vi "MeasureEQE_ActiveX.vi"(6 "Skip?":bool, 8 "error in (no error)":errorcluster, 9 "Save data file path":string, 10 "Scan settings":T1={"J-V scan"=TRUE, "J-t scan"=FALSE, "Min voltage (V)"=0.0, "Max voltage (V)"=1.4, "Step (V)"=0.01, "Measurement delay (ms)"=10.0, "1st scan FB-SC"=TRUE, "Inverted structure"=FALSE, "Stabilisation time (s)"=0.0, "Stabilisation mode"=0, "Stabilisation value (V or A) "=0.0, "Step time (s)"=1.0, "Integration time"=0, "Repeat light scans"=FALSE, "Stabilisation in the dark?"=FALSE, "J-t Min (V)"=0.0, "J-t Max (V)"=1.4, "J-t Step (V)"=0.01, "Max. power stabilisation"=FALSE, "J-t 1st scan FB-SC"=TRUE, "J-t Inverted structure"=FALSE, "Max power tracking"=FALSE, "Vmp (V)"=0.7, "Total stabilisation time (s)"=100.0, "J-t best pixel only"=0, "Max power best pixel only"=0, "Vmp from J-V scan"=FALSE, "Intensity dependence"=FALSE, "P dep best pixel only"=0, "External quantum efficiency"=FALSE, "EQE best pixel only"=0, "WL min (nm)"=300.0, "WL max (nm)"=900.0, "WL step (nm)"=5.0, "Wait (ms)"=100.0, "No. of repeat scans"=2.0, "Only repeat for best pixel"=0, "Chopper Freq.  (Hz)"=90.0, "Time Constant (s)"=2.0, "Stabilisation time step (s)"=1.0, "Illumination conditions"=2, "Scan rate min (V/s)"=0.1, "Scan rate max (V/s)"=1.0, "No. of scan rate steps"=1.0, "Scan rate voltage step priority"=FALSE, "Scan rate measurement delay priority"=FALSE, "J-t Illumination conditions"=0, "White bias  (no. of suns)"=200.0, "Max P stab. Specific voltage"=FALSE} {"J-t Illumination conditions" items=["Light only", "Dark only", "Light then dark", "Dark then light"]; "No. of scan rate steps" min=1.0 step=1.0; "Illumination conditions" items=["Light only", "Dark only", "Light then dark", "Dark then light", "Light then dark then light", "Dark then light then dark"]; "Time Constant (s)" items=["0.003", "0.01", "0.03", "0.1", "0.3", "1", "3", "10", "30", "100"]; "Only repeat for best pixel" items=["only for best pixel", "for best 2 pixels", "for best 3 pixels", "for best 4 pixels", "for best 5 pixels", "for best 6 pixels", "for best 7 pixels", "for all pixels"]; "No. of repeat scans" min=1.0 step=1.0; "EQE best pixel only" items=["only the best pixel", "the best 2 pixel", "the best 3 pixel", "the best 4 pixel", "the best 5 pixel", "the best 6 pixel", "the best 7 pixel", "all pixels"]; "P dep best pixel only" items=["only the best pixel", "the best 2 pixels", "the best 3 pixels", "the best 4 pixels", "the best 5 pixels", "the best 6 pixels", "the best 7 pixels", "all pixels"]; "Max power best pixel only" items=["only the best pixel", "the best 2 pixels", "the best 3 pixels", "the best 4 pixels", "the best 5 pixels", "the best 6 pixels", "the best 7 pixels", "all pixels"]; "J-t best pixel only" items=["only the best pixel", "the best 2 pixels", "the best 3 pixels", "the best 4 pixels", "the best 5 pixels", "the best 6 pixels", "the best 7 pixels", "all pixels"]; "Integration time" items=["Fast", "Normal", "High Accuracy"]; "Stabilisation mode" items=["V", "I"]; "Measurement delay (ms)" min=10.0}) -> (0 "error out":errorcluster, 1 "Min WL (nm)":string, 2 "Max WL (nm)":string, 3 "EQE data file path":path)   [LabVIEW 2011]
uses:
  TypeDefs/Scan settings.ctl
  TypeDefs/Settings Boolean.ctl
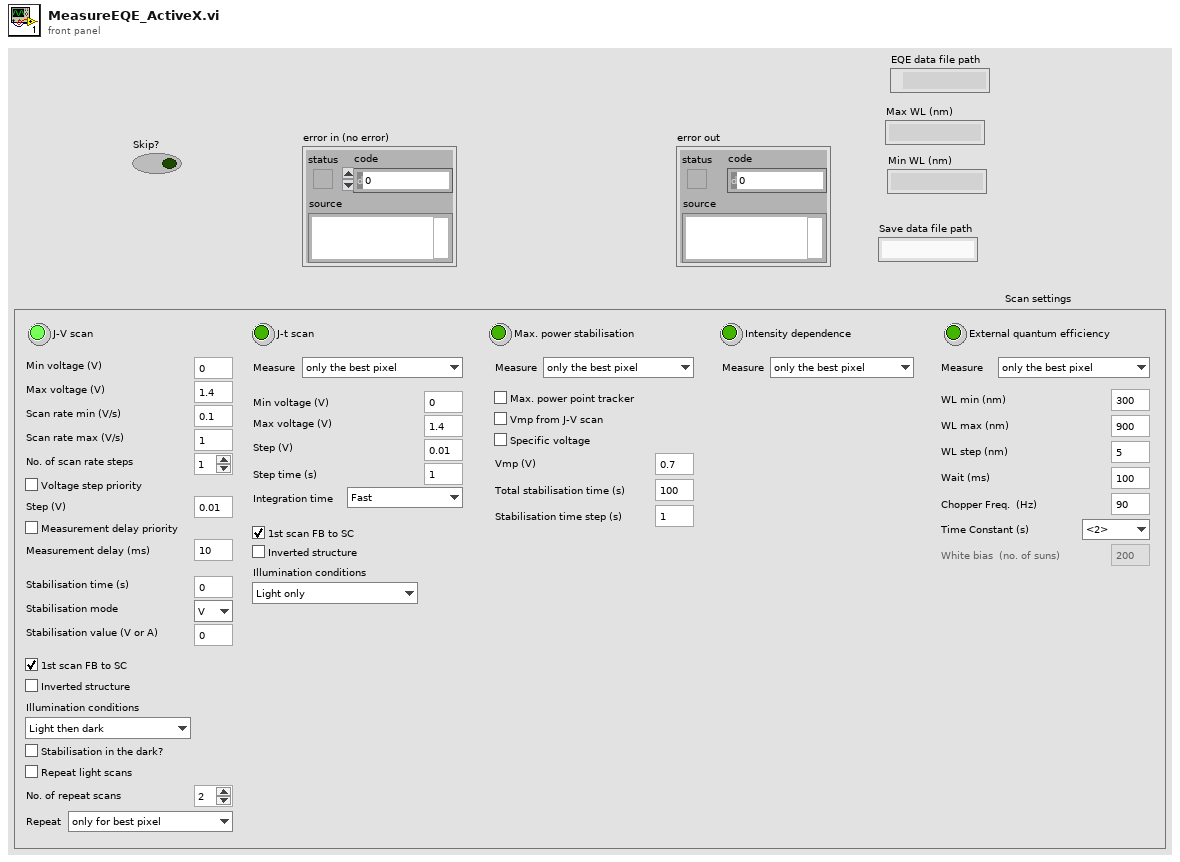
[diagram p1: front panel]
types:
  T1 = typedef "Scan settings.ctl" = cluster{"J-V scan":T2, "J-t scan":bool, "Min voltage (V)":dbl, "Max voltage (V)":dbl, "Step (V)":dbl, "Measurement delay (ms)":dbl, "1st scan FB-SC":bool, "Inverted structure":bool, "Stabilisation time (s)":dbl, "Stabilisation mode":u16, "Stabilisation value (V or A) ":dbl, "Step time (s)":dbl, "Integration time":u16, "Repeat light scans":bool, "Stabilisation in the dark?":bool, "J-t Min (V)":dbl, "J-t Max (V)":dbl, "J-t Step (V)":dbl, "Max. power stabilisation":bool, "J-t 1st scan FB-SC":bool, "J-t Inverted structure":bool, "Max power tracking":bool, "Vmp (V)":dbl, "Total stabilisation time (s)":dbl, "J-t best pixel only":u16, "Max power best pixel only":u16, "Vmp from J-V scan":bool, "Intensity dependence":bool, "P dep best pixel only":u16, "External quantum efficiency":bool, "EQE best pixel only":u16, "WL min (nm)":dbl, "WL max (nm)":dbl, "WL step (nm)":dbl, "Wait (ms)":dbl, "No. of repeat scans":dbl, "Only repeat for best pixel":u16, "Chopper Freq.  (Hz)":dbl, "Time Constant (s)":dbl, "Stabilisation time step (s)":dbl, "Illumination conditions":u16, "Scan rate min (V/s)":dbl, "Scan rate max (V/s)":dbl, "No. of scan rate steps":dbl, "Scan rate voltage step priority":bool, "Scan rate measurement delay priority":bool, "J-t Illumination conditions":u16, "White bias  (no. of suns)":dbl, "Max P stab. Specific voltage":bool}
  T2 = typedef "Settings Boolean.ctl" = bool
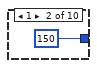
[diagram p2: hidden frame]
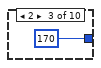
[diagram p3: hidden frame]
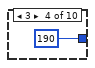
[diagram p4: hidden frame]
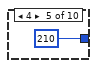
[diagram p5: hidden frame]
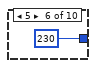
[diagram p6: hidden frame]
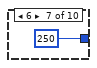
[diagram p7: hidden frame]
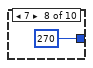
[diagram p8: hidden frame]
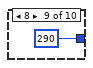
[diagram p9: hidden frame]
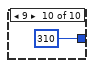
[diagram p10: hidden frame]
diagram:
  n1 = case shown="False" "Skip?" {
    tunnel: "error in (no error)" -> [w273 w285]
    tunnel: [w4 w285] -> w2
    frame False {
      w13 = 2000.0  # Buffer (ms)
      w14 = 11000.0  # Grating change time (ms)
      w17 = 2000.0  # Filter change time (ms)
      w18 = 22000.0  # initialisation time (ms)
      w21 = 1150.0  # time to change wl and measure (ms)
      # "click \"Clear graph\""
      # "click \"Ok\""
      # "Save file"
      # "click \"Save scan data\""
      # "click \"File\""
      # "click \"Take a simple wavelength scan\""
      # "click \"Scan\""
      # "Click \"OK\""
      # "Set wait"
      # "Set wavlength step"
      # "Set end wavlength"
      # "Set start wavlength"
      # "click \"Click Setup Scan Wavelength Parameters\""
      # "click \"Scan\""
      # "click \"OK\""
      # "click \"AC\""
      # "click \"Ref Type\""
      # "set chopper frequency (Hz)"
      # "choose time constant"
      # "click \"Time Constant\""
      # "click \"CHANNEL 2\""
      # "click \"Channel Setup\""
      # "click \"Setup Parameters\""
      # "click \"Detector\""
      n2 = Automation Open(error in (no error)=w273, Automation Refnum=refnum<k7> refnum ("AutoItX3Lib.IAutoItX3")) -> (Automation Refnum=w238:refnum<k7>, error out=w237:errorcluster)  [unwired: 2 in]
      n3 = invoke class="IAutoItX3" method="WinActivate"(reference=w238, error in=w237, "strTitle"="Newport Oriel Tracq Basic Version 6.2", "strText"="") -> (reference out=w272:refnum<k7>, error out=w265:errorcluster)  [unwired: 1 in, 3 out]
      n4 = invoke class="IAutoItX3" method="WinWaitActive"(reference=w272, error in=w265, "strTitle"="Newport Oriel Tracq Basic Version 6.2", "strText"="", "nTimeout"=2000) -> (reference out=w266:refnum<k7>, error out=w264:errorcluster)  [unwired: 1 in, 4 out]
      n5 = invoke class="IAutoItX3" method="MouseClick"(reference=w266, error in=w264, "strButton"="primary", "nX"=250, "nY"=40, "nClicks"=1) -> (reference out=w258:refnum<k7>, error out=w257:errorcluster)  [unwired: 2 in, 6 out]
      n6 = invoke class="IAutoItX3" method="Sleep"(reference=w258, error in=w257, "nMilliseconds"=100) -> (reference out=w252:refnum<k7>, error out=w251:errorcluster)  [unwired: 1 in, 2 out]
      n7 = invoke class="IAutoItX3" method="MouseClick"(reference=w252, error in=w251, "strButton"="primary", "nX"=290, "nY"=90, "nClicks"=1) -> (reference out=w247:refnum<k7>, error out=w246:errorcluster)  [unwired: 2 in, 6 out]
      n8 = invoke class="IAutoItX3" method="WinWaitActive"(reference=w247, error in=w246, "strTitle"="Merlin Setup", "strText"="", "nTimeout"=5000) -> (reference out=w232:refnum<k7>, error out=w231:errorcluster)  [unwired: 1 in, 4 out]
      n9 = invoke class="IAutoItX3" method="MouseClick"(reference=w232, error in=w231, "strButton"="primary", "nX"=450, "nY"=70, "nClicks"=1) -> (reference out=w223:refnum<k7>, error out=w222:errorcluster)  [unwired: 2 in, 6 out]
      n10 = invoke class="IAutoItX3" method="Sleep"(reference=w223, error in=w222, "nMilliseconds"=100) -> (reference out=w225:refnum<k7>, error out=w224:errorcluster)  [unwired: 1 in, 2 out]
      n11 = invoke class="IAutoItX3" method="MouseClick"(reference=w225, error in=w224, "strButton"="primary", "nX"=365, "nY"=140, "nClicks"=1) -> (reference out=w214:refnum<k7>, error out=w213:errorcluster)  [unwired: 2 in, 6 out]
      n12 = invoke class="IAutoItX3" method="Sleep"(reference=w214, error in=w213, "nMilliseconds"=100) -> (reference out=w216:refnum<k7>, error out=w215:errorcluster)  [unwired: 1 in, 2 out]
      n13 = Unbundle By Name("Scan settings") -> ("WL min (nm)"=w11:dbl, "WL max (nm)"=w12:dbl, "WL step (nm)"=w10:dbl, "Wait (ms)"=w9:dbl, "Chopper Freq.  (Hz)"=w30:dbl, "Time Constant (s)"=w33:dbl)
      n14 = invoke class="IAutoItX3" method="MouseClick"(reference=w216, error in=w215, "strButton"="primary", "nX"=865, "nY"=310, "nClicks"=1) -> (reference out=w211:refnum<k7>, error out=w210:errorcluster)  [unwired: 2 in, 6 out]
      n15 = case shown="0, Default" w33 {
        tunnel: [130 150 170 190 210 230 250 270 290 310] -> w31
        frame 0, Default {
        }
        frame 1 {
        }
        frame 2 {
        }
        frame 3 {
        }
        frame 4 {
        }
        frame 5 {
        }
        frame 6 {
        }
        frame 7 {
        }
        frame 8 {
        }
        frame 9 {
        }
      }
      n16 = invoke class="IAutoItX3" method="Sleep"(reference=w211, error in=w210, "nMilliseconds"=100) -> (reference out=w204:refnum<k7>, error out=w203:errorcluster)  [unwired: 1 in, 2 out]
      n17 = invoke class="IAutoItX3" method="MouseClick"(reference=w204, error in=w203, "strButton"="primary", "nX"=865, "nY"=w31, "nClicks"=1) -> (reference out=w206:refnum<k7>, error out=w205:errorcluster)  [unwired: 2 in, 6 out]
      n18 = Number To Fractional String(number=w11) -> (F-format string=w28:string)  [unwired: 3 in]
      "Min WL (nm)" <- w28
      n19 = Number To Fractional String(number=w12) -> (F-format string=w27:string)  [unwired: 3 in]
      "Max WL (nm)" <- w27
      n20 = Number To Fractional String(number=w10) -> (F-format string=w26:string)  [unwired: 3 in]
      n21 = Number To Fractional String(number=w9) -> (F-format string=w25:string)  [unwired: 3 in]
      n22 = Number To Fractional String(number=w30) -> (F-format string=w29:string)  [unwired: 3 in]
      n23 = invoke class="IAutoItX3" method="Sleep"(reference=w206, error in=w205, "nMilliseconds"=100) -> (reference out=w202:refnum<k7>, error out=w201:errorcluster)  [unwired: 1 in, 2 out]
      n24 = Subtract(x=w12, y=w11) -> (x-y=w24:dbl)
      n25 = Divide(x=w24, y=w10) -> (x/y=w23:dbl)
      n26 = Increment(x=w23) -> (x+1=w22:dbl)
      n27 = Add(x=w9, y=w21) -> (x+y=w20:dbl)
      n28 = Multiply(x=w22, y=w20) -> (x*y=w19:dbl)
      n29 = invoke class="IAutoItX3" method="MouseClickDrag"(reference=w202, error in=w201, "strButton"="primary", "nX1"=870 ("nX"), "nY1"=370 ("nY"), "nX2"=825 ("nClicks"), "nY2"=370 ("nClicks")) -> (reference out=w240:refnum<k7>, error out=w239:errorcluster)  [unwired: 2 in, 7 out]
      n30 = Multiply(x=w17, y=2.0) -> (x*y=w15:dbl)
      n31 = invoke class="IAutoItX3" method="Send"(reference=w240, error in=w239, "strSendText"=w29) -> (reference out=w193:refnum<k7>, error out=w192:errorcluster)  [unwired: 2 in, 3 out]
      n32 = Compound Arithmetic op=ADD(w19, w18, w15, w14, w13) -> (w8:dbl)
      n33 = invoke class="IAutoItX3" method="Sleep"(reference=w193, error in=w192, "nMilliseconds"=100) -> (reference out=w195:refnum<k7>, error out=w194:errorcluster)  [unwired: 1 in, 2 out]
      n34 = To Long Integer(number=w8) -> (32bit integer=w7:i32)
      n35 = invoke class="IAutoItX3" method="MouseClick"(reference=w195, error in=w194, "strButton"="primary", "nX"=910, "nY"=695, "nClicks"=1) -> (reference out=w184:refnum<k7>, error out=w183:errorcluster)  [unwired: 2 in, 6 out]
      n36 = invoke class="IAutoItX3" method="Sleep"(reference=w184, error in=w183, "nMilliseconds"=100) -> (reference out=w186:refnum<k7>, error out=w185:errorcluster)  [unwired: 1 in, 2 out]
      n37 = invoke class="IAutoItX3" method="MouseClick"(reference=w186, error in=w185, "strButton"="primary", "nX"=830, "nY"=740, "nClicks"=1) -> (reference out=w175:refnum<k7>, error out=w174:errorcluster)  [unwired: 2 in, 6 out]
      n38 = invoke class="IAutoItX3" method="Sleep"(reference=w175, error in=w174, "nMilliseconds"=100) -> (reference out=w177:refnum<k7>, error out=w176:errorcluster)  [unwired: 1 in, 2 out]
      n39 = invoke class="IAutoItX3" method="MouseClick"(reference=w177, error in=w176, "strButton"="primary", "nX"=1125, "nY"=75, "nClicks"=1) -> (reference out=w170:refnum<k7>, error out=w169:errorcluster)  [unwired: 2 in, 6 out]
      n40 = invoke class="IAutoItX3" method="WinWaitActive"(reference=w170, error in=w169, "strTitle"="Newport Oriel Tracq Basic Version 6.2", "strText"="", "nTimeout"=10000) -> (reference out=w155:refnum<k7>, error out=w154:errorcluster)  [unwired: 1 in, 4 out]
      n41 = invoke class="IAutoItX3" method="MouseClick"(reference=w155, error in=w154, "strButton"="primary", "nX"=50, "nY"=35, "nClicks"=1) -> (reference out=w157:refnum<k7>, error out=w156:errorcluster)  [unwired: 2 in, 6 out]
      n42 = invoke class="IAutoItX3" method="Sleep"(reference=w157, error in=w156, "nMilliseconds"=100) -> (reference out=w159:refnum<k7>, error out=w158:errorcluster)  [unwired: 1 in, 2 out]
      n43 = invoke class="IAutoItX3" method="MouseClick"(reference=w159, error in=w158, "strButton"="primary", "nX"=45, "nY"=55, "nClicks"=1) -> (reference out=w150:refnum<k7>, error out=w149:errorcluster)  [unwired: 2 in, 6 out]
      n44 = invoke class="IAutoItX3" method="WinWaitActive"(reference=w150, error in=w149, "strTitle"="Enter Scan Parameters", "strText"="", "nTimeout"=2000) -> (reference out=w141:refnum<k7>, error out=w140:errorcluster)  [unwired: 1 in, 4 out]
      n45 = invoke class="IAutoItX3" method="MouseClickDrag"(reference=w141, error in=w140, "strButton"="primary", "nX1"=675 ("nX"), "nY1"=470 ("nY"), "nX2"=600 ("nClicks"), "nY2"=470 ("nClicks")) -> (reference out=w143:refnum<k7>, error out=w142:errorcluster)  [unwired: 2 in, 7 out]
      n46 = invoke class="IAutoItX3" method="Send"(reference=w143, error in=w142, "strSendText"=w28) -> (reference out=w132:refnum<k7>, error out=w131:errorcluster)  [unwired: 2 in, 3 out]
      n47 = invoke class="IAutoItX3" method="MouseClickDrag"(reference=w132, error in=w131, "strButton"="primary", "nX1"=675 ("nX"), "nY1"=515 ("nY"), "nX2"=600 ("nClicks"), "nY2"=515 ("nClicks")) -> (reference out=w134:refnum<k7>, error out=w133:errorcluster)  [unwired: 2 in, 7 out]
      n48 = invoke class="IAutoItX3" method="Send"(reference=w134, error in=w133, "strSendText"=w27) -> (reference out=w123:refnum<k7>, error out=w122:errorcluster)  [unwired: 2 in, 3 out]
      n49 = invoke class="IAutoItX3" method="MouseClickDrag"(reference=w123, error in=w122, "strButton"="primary", "nX1"=675 ("nX"), "nY1"=560 ("nY"), "nX2"=600 ("nClicks"), "nY2"=560 ("nClicks")) -> (reference out=w125:refnum<k7>, error out=w124:errorcluster)  [unwired: 2 in, 7 out]
      n50 = invoke class="IAutoItX3" method="Send"(reference=w125, error in=w124, "strSendText"=w26) -> (reference out=w114:refnum<k7>, error out=w113:errorcluster)  [unwired: 2 in, 3 out]
      n51 = invoke class="IAutoItX3" method="MouseClickDrag"(reference=w114, error in=w113, "strButton"="primary", "nX1"=675 ("nX"), "nY1"=600 ("nY"), "nX2"=600 ("nClicks"), "nY2"=600 ("nClicks")) -> (reference out=w116:refnum<k7>, error out=w115:errorcluster)  [unwired: 2 in, 7 out]
      n52 = invoke class="IAutoItX3" method="Send"(reference=w116, error in=w115, "strSendText"=w25) -> (reference out=w103:refnum<k7>, error out=w102:errorcluster)  [unwired: 2 in, 3 out]
      n53 = invoke class="IAutoItX3" method="MouseClick"(reference=w103, error in=w102, "strButton"="primary", "nX"=801, "nY"=425, "nClicks"=1) -> (reference out=w105:refnum<k7>, error out=w104:errorcluster)  [unwired: 2 in, 6 out]
      n54 = invoke class="IAutoItX3" method="WinWaitActive"(reference=w105, error in=w104, "strTitle"="Newport Oriel Tracq Basic Version 6.2", "strText"="", "nTimeout"=2000) -> (reference out=w94:refnum<k7>, error out=w93:errorcluster)  [unwired: 1 in, 4 out]
      n55 = invoke class="IAutoItX3" method="MouseClick"(reference=w94, error in=w93, "strButton"="primary", "nX"=50, "nY"=35, "nClicks"=1) -> (reference out=w96:refnum<k7>, error out=w95:errorcluster)  [unwired: 2 in, 6 out]
      n56 = invoke class="IAutoItX3" method="Sleep"(reference=w96, error in=w95, "nMilliseconds"=100) -> (reference out=w86:refnum<k7>, error out=w85:errorcluster)  [unwired: 1 in, 2 out]
      n57 = invoke class="IAutoItX3" method="MouseClick"(reference=w86, error in=w85, "strButton"="primary", "nX"=60, "nY"=80, "nClicks"=1) -> (reference out=w88:refnum<k7>, error out=w87:errorcluster)  [unwired: 2 in, 6 out]
      n58 = invoke class="IAutoItX3" method="Sleep"(reference=w88, error in=w87, "nMilliseconds"=w7) -> (reference out=w71:refnum<k7>, error out=w70:errorcluster)  [unwired: 1 in, 2 out]
      n59 = invoke class="IAutoItX3" method="MouseClick"(reference=w71, error in=w70, "strButton"="primary", "nX"=15, "nY"=35, "nClicks"=1) -> (reference out=w79:refnum<k7>, error out=w78:errorcluster)  [unwired: 2 in, 6 out]
      n60 = invoke class="IAutoItX3" method="Sleep"(reference=w79, error in=w78, "nMilliseconds"=100) -> (reference out=w73:refnum<k7>, error out=w72:errorcluster)  [unwired: 1 in, 2 out]
      n61 = invoke class="IAutoItX3" method="MouseClick"(reference=w73, error in=w72, "strButton"="primary", "nX"=30, "nY"=75, "nClicks"=1) -> (reference out=w66:refnum<k7>, error out=w65:errorcluster)  [unwired: 2 in, 6 out]
      n62 = invoke class="IAutoItX3" method="WinWaitActive"(reference=w66, error in=w65, "strTitle"="Choose file to write.", "strText"="", "nTimeout"=2000) -> (reference out=w55:refnum<k7>, error out=w54:errorcluster)  [unwired: 1 in, 4 out]
      n63 = String To Path(string="Save data file path") -> (path=→"EQE data file path":path)
      n64 = invoke class="IAutoItX3" method="Send"(reference=w55, error in=w54, "strSendText"="Save data file path") -> (reference out=w53:refnum<k7>, error out=w52:errorcluster)  [unwired: 2 in, 3 out]
      n65 = invoke class="IAutoItX3" method="MouseClick"(reference=w53, error in=w52, "strButton"="primary", "nX"=880, "nY"=700, "nClicks"=1) -> (reference out=w57:refnum<k7>, error out=w56:errorcluster)  [unwired: 2 in, 6 out]
      n66 = invoke class="IAutoItX3" method="WinWaitActive"(reference=w57, error in=w56, "strTitle"="Newport Oriel Tracq Basic Version 6.2", "strText"="", "nTimeout"=2000) -> (reference out=w47:refnum<k7>, error out=w46:errorcluster)  [unwired: 1 in, 4 out]
      n67 = invoke class="IAutoItX3" method="MouseClick"(reference=w47, error in=w46, "strButton"="primary", "nX"=1060, "nY"=115, "nClicks"=1) -> (reference out=w38:refnum<k7>, error out=w37:errorcluster)  [unwired: 2 in, 6 out]
      n68 = invoke class="IAutoItX3" method="WinActivate"(reference=w38, error in=w37, "strTitle"="Automated JV Measurement.vi", "strText"="") -> (reference out=w45:refnum<k7>, error out=w39:errorcluster)  [unwired: 1 in, 3 out]
      n69 = invoke class="IAutoItX3" method="WinWaitActive"(reference=w45, error in=w39, "strTitle"="Automated JV Measurement.vi", "strText"="", "nTimeout"=2000) -> (reference out=w36:refnum<k7>, error out=w35:errorcluster)  [unwired: 1 in, 4 out]
      n70 = Close Reference(reference=w36, error in (no error)=w35) -> (error out=w4:errorcluster)
    }
    frame True {
    }
  }
  "error out" <- w2
